vi "MC - Read INI.vi"(0 "INI Name":string) -> (2 "INI Array":string[][][](array[string]), 3 "error out":errorcluster)   [LabVIEW 2015]
uses:
  <vilib>/Utility/config.llb/Read Key (String).vi
  <vilib>/Utility/config.llb/NI_LVConfig.lvlib
panel:
  in  "Case Constant\n(See Context Help)":string="Don't Run"
  out "No. of Keys per Section":i32[](array[numeric])
  out "INI path":path
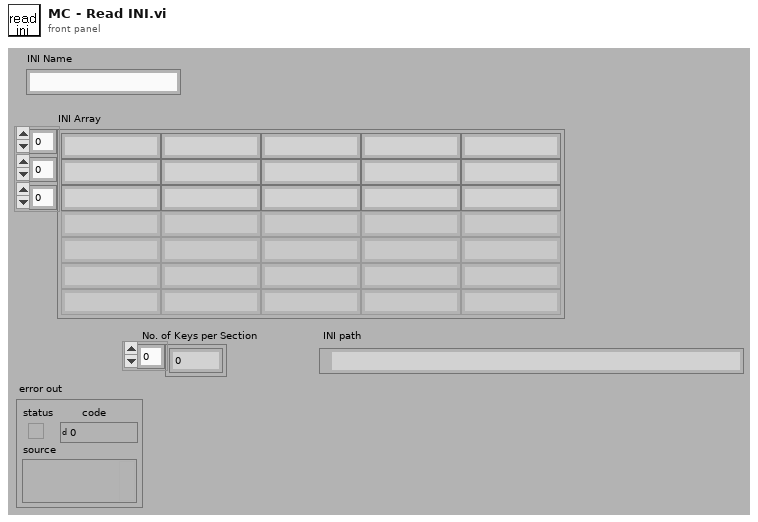
[diagram p1: front panel]
types:
  T1 = typedef "NI_LVConfig.lvlib/Config Data RefNum.ctl" = refnum<k1>
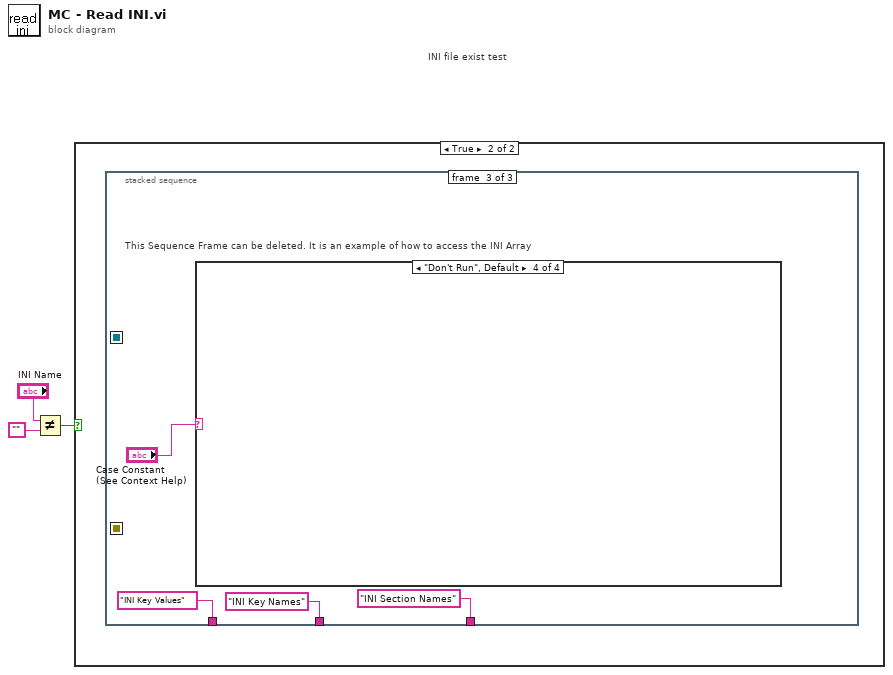
[diagram p0: block diagram]
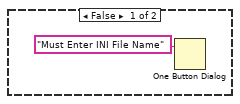
[diagram p2: hidden frame]
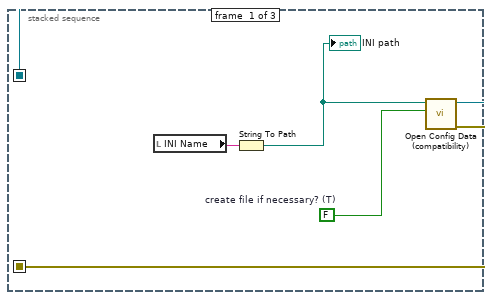
[diagram p3: hidden frame]
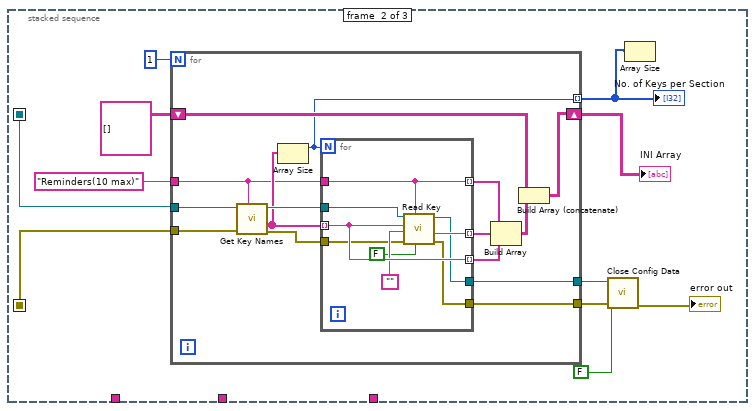
[diagram p4: hidden frame]
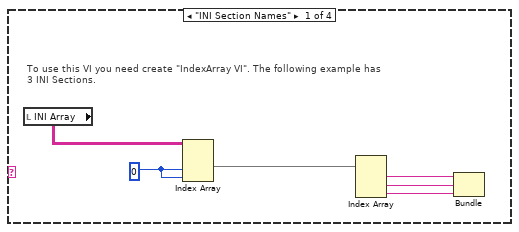
[diagram p5: hidden frame]
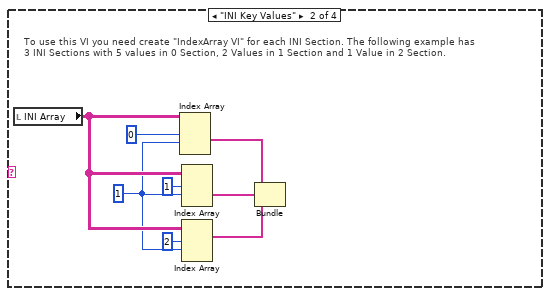
[diagram p6: hidden frame]
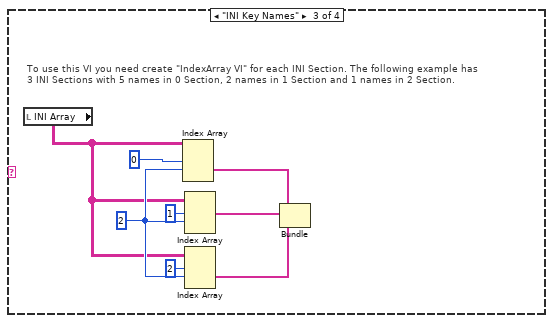
[diagram p7: hidden frame]
diagram:
  # "INI file exist test"
  n1 = Not Equal?(x="INI Name", y="") -> (x != y?=w3:bool)
  n2 = case shown="True" w3 {
    frame False {
      n3 = One Button Dialog(message="Must Enter INI File Name") -> ()  [unwired: 2 out]
    }
    frame True {
      n4 = stacked-sequence {
        seq-local: [w9 _ _] -> [_ w13 _]
        seq-local: [w7 _ _] -> [_ w12 _]
        tunnel: [_ _ "INI Section Names"] -> _
        tunnel: [_ _ "INI Key Names"] -> _
        tunnel: [_ _ "INI Key Values"] -> _
        frame #0 {
          w8 = FALSE  # create file if necessary? (T)
          n5 = local read "INI Name"() -> (w6:string)
          n6 = String To Path(string=w6) -> (path=w5:path)
          "INI path" <- w5
          n7 = call <vilib>:"Open Config Data (compatibility).vi"("create file if necessary (T)"=w8, "configuration file path"=w5) -> ("error out"=w7:errorcluster, "refnum"=w9:T1)  [unwired: 7 in, 1 out]
        }
        frame #1 {
          n8 = for {
            N: 1 -> [_]
            tunnel: "Reminders(10 max)" -> [w21]
            shift-right: [w33] -> w19
            shift-left: string[][][] [] -> [w32]
            tunnel: w13 -> [w31]
            tunnel: [w26] -> w18 mode=indexing
            tunnel: w12 -> [w25]
            tunnel: [w23] -> w17
            tunnel: [w22] -> w16
            n9 = call <vilib>:"Get Key Names.vi"("section"=w21, "error in (no error)"=w25, "refnum"=w31) -> ("error out"=w24:errorcluster, "key names"=w29:string[], "refnum out"=w30:T1)  [unwired: 6 out]
            n10 = Array Size(array=w29) -> (size(s)=w26:i32)
            n11 = for {
              N: w26 -> [_]
              tunnel: w29 -> [w44] mode=indexing
              tunnel: w21 -> [w43]
              tunnel: [w44] -> w27 mode=indexing
              tunnel: [w43] -> w35 mode=indexing
              tunnel: [w42] -> w28 mode=indexing
              tunnel: w30 -> [w40]
              tunnel: w24 -> [w39]
              tunnel: [w38] -> w23
              tunnel: [w37] -> w22
              n12 = call-poly <vilib>:"Read Key.vi"("read raw string? (F)"=FALSE, "section"=w43, "error in (no error)"=w39, "default value"="", "key"=w44, "refnum"=w40) -> ("error out"=w37:errorcluster, "value"=w42:string, "refnum out"=w38:T1)  [unwired: 3 out]
            }
            n13 = Build Array(w35, w28, w27) -> (w34:string[][])
            n14 = Build Array (concatenate)(w32, w34) -> (w33:string[][][])
          }
          "INI Array" <- w19
          "No. of Keys per Section" <- w18
          n15 = call <vilib>:"Close Config Data.vi"("error in (no error)"=w16, "write file if changed (T)"=FALSE ("write configuration file? (T)"), "refnum"=w17) -> ("error out"=→"error out":errorcluster)  [unwired: 8 out]
          n16 = Array Size(array=w18) -> ()  [unwired: 1 out]
        }
        frame #2 {
          # "This Sequence Frame can be deleted. It is an example of how to access the INI Array"
          n17 = case shown="\"Don't Run\", Default" "Case Constant\n(See Context Help)" {
            frame "INI Section Names" {
              w49 = 0 ("Index (page)")
              # "To use this VI you need create \"IndexArray VI\". The following example has\n3 INI Sections."
              n18 = local read "INI Array"() -> (w50:string[][][])
              n19 = Index Array(array=w50, index (dim 1)=w49, index (dim 2)=w49) -> (element=w51:string[])  [unwired: 1 in]
              n20 = Index Array(array=w51) -> (element #1=w54:string, element #2=w52:string, element #3=w53:string)  [unwired: 3 in]
              n21 = Bundle("String"=w54, "String"=w52, "String"=w53) -> ()  [unwired: 2 out]
            }
            frame "INI Key Values" {
              w58 = 1 ("Disabled Index (row)")
              # "To use this VI you need create \"IndexArray VI\" for each INI Section. The following example has\n3 INI Sections with 5 values in 0 Section, 2 Values in 1 Section and 1 Value in 2 Section."
              n22 = local read "INI Array"() -> (w60:string[][][])
              n23 = Index Array(array=w60, index (dim 0)=0 ("Index (page)"), index (dim 1)=w58) -> (element=w57:string[])  [unwired: 1 in]
              n24 = Index Array(array=w60, index (dim 0)=1 ("Index (page)"), index (dim 1)=w58) -> (element=w56:string[])  [unwired: 1 in]
              n25 = Index Array(array=w60, index (dim 0)=2 ("Index (page)"), index (dim 1)=w58) -> (element=w55:string[])  [unwired: 1 in]
              n26 = Bundle("INI Array"=w57, "INI Array"=w56, "INI Array"=w55) -> ()  [unwired: 2 out]
            }
            frame "INI Key Names" {
              w67 = 2 ("Disabled Index (row)")
              # "To use this VI you need create \"IndexArray VI\" for each INI Section. The following example has\n3 INI Sections with 5 names in 0 Section, 2 names in 1 Section and 1 names in 2 Section."
              n27 = local read "INI Array"() -> (w66:string[][][])
              n28 = Index Array(array=w66, index (dim 0)=0 ("Index (page)"), index (dim 1)=w67) -> (element=w65:string[])  [unwired: 1 in]
              n29 = Index Array(array=w66, index (dim 0)=1 ("Index (page)"), index (dim 1)=w67) -> (element=w63:string[])  [unwired: 1 in]
              n30 = Index Array(array=w66, index (dim 0)=2 ("Index (page)"), index (dim 1)=w67) -> (element=w64:string[])  [unwired: 1 in]
              n31 = Bundle("INI Array"=w63, "INI Array"=w65, "INI Array"=w64) -> ()  [unwired: 2 out]
            }
            frame "Don't Run", Default {
            }
          }
        }
      }
    }
  }
